vi "Segmentation.vi"(9 "sample time":dbl=1000.0, 11 "relative time":dbl[](array[numeric])=[1.0, 4.0, 7.0, 12.0, 15.0, 20.0, 31.0, 48.0, 59.0, 67.0, 96.0, 105.0, 121.0, 143.0, 144.0, 159.0, 171.0, 179.0, 185.0, 246.0] format="%#_10g") -> (1 "Segmentation":sgl[](array[numeric]), 2 "mean":dbl format="%0.2f", 3 "tau":dbl[](array[numeric]) format="%#_10g")   [LabVIEW 2015]
uses:
  <vilib>/Analysis/baseanly.llb/Mean (DBL).vi
  <vilib>/Analysis/NI_AALBase.lvlib
panel:
  out "Size in":i32
  out "index":sgl format="%#_10g"
  out "size segmentation":i32
  out "size tau":i32
  out "vector size":i32
  out "LsupLazo":sgl format="%#_10g"
  out "Datolazo":dbl format="%#_10g"
  out "Lsup":dbl format="%#_10g"
  out "dato":dbl format="%#_10g"
  out "Linf":dbl format="%#_10g"
  out "i vector":i32
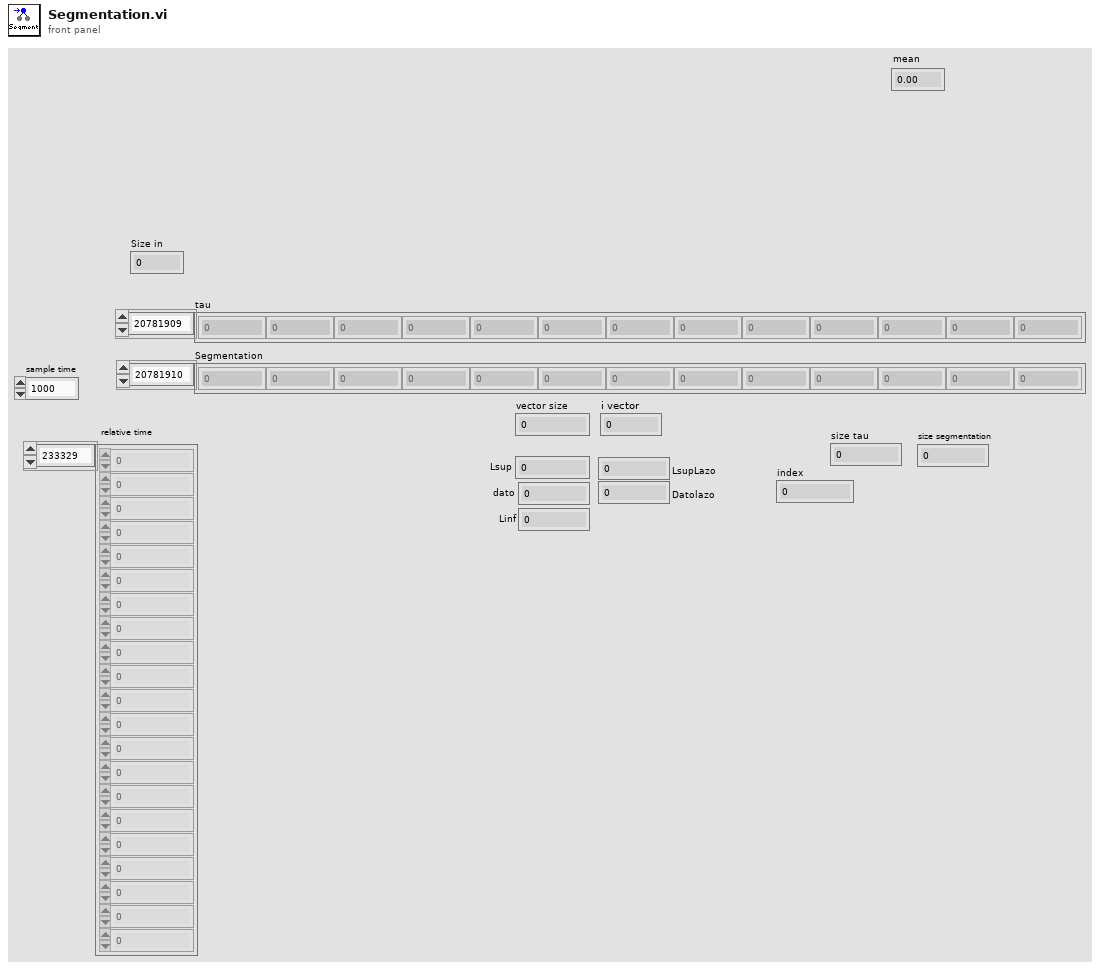
[diagram p1: front panel]
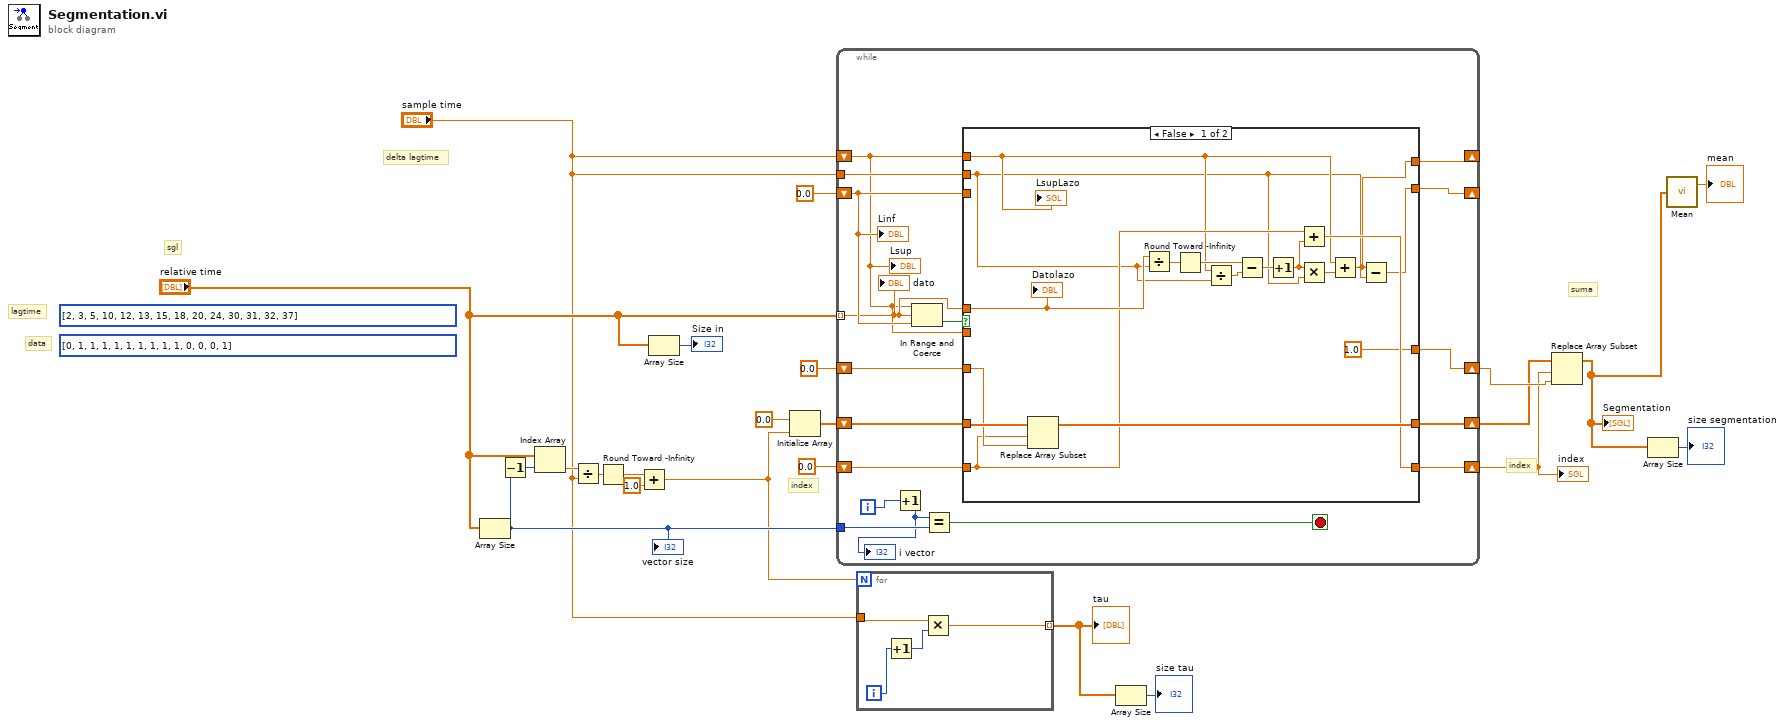
[diagram p0: block diagram]
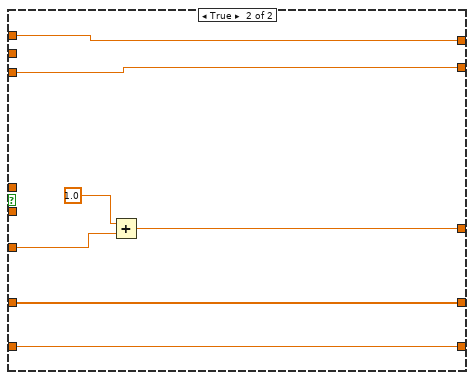
[diagram p2: hidden frame]
diagram:
  (unwired) i32[] [0, 1, 1, 1, 1, 1, 1, 1, 1, 1, 0, 0, 0, 1]
  (unwired) i32[] [2, 3, 5, 10, 12, 13, 15, 18, 20, 24, 30, 31, 32, 37]
  # "sgl"
  # "suma"
  # "index"
  # "index"
  # "delta lagtime"
  # "data"
  # "lagtime"
  n1 = Array Size(array="relative time") -> (size(s)=w18:i32)
  "vector size" <- w18
  n2 = Decrement(x=w18) -> (x-1=w16:i32)
  n3 = Index Array(array="relative time", index=w16) -> (element=w15:dbl)
  n4 = Divide(x=w15, y="sample time") -> (x/y=w19:dbl)
  n5 = Round Toward -Infinity(1:w19) -> (0:w14:dbl)
  n6 = Add(x=w14, y=sgl 1.0) -> (x+y=w12:dbl)
  n7 = Array Size(array="relative time") -> (size(s)=→"Size in":i32)
  n8 = Initialize Array(sgl 0.0 ("lower limit"), w12) -> (w21:sgl[])
  n9 = while {
    tunnel: "relative time" -> [w31] mode=indexing
    shift-right: [w26] -> w8
    shift-left: sgl 0.0 ("lower limit") -> [w39]
    shift-right: [w30] -> _
    shift-left: "sample time" -> [w28]
    tunnel: "sample time" -> [w29]
    shift-right: [w37] -> _
    shift-left: sgl 0.0 ("lower limit") -> [w38]
    tunnel: w18 -> [w36]
    shift-right: [w32] -> w6
    shift-left: w21 -> [w35]
    shift-right: [w33] -> w7
    shift-left: sgl 0.0 ("lower limit") -> [w34]
    i -> [w25]
    stop <- w27 stop-if-true
    n10 = Increment(x=w25) -> (x+1=w24:i32)
    "i vector" <- w24
    n11 = In Range and Coerce(upper limit=w28, x=w31, lower limit=w38) -> (In Range?=w40:bool)  [unwired: 1 out]
    n12 = Equal?(x=w24, y=w36) -> (x = y?=w27:bool)
    n13 = case shown="False" w40 {
      tunnel: [sgl 1.0 ("lower limit") w60] -> w26
      tunnel: w39 -> [w56 w64]
      tunnel: w28 -> [w46 w63]
      tunnel: [w44 w63] -> w30
      tunnel: w29 -> [w43 _]
      tunnel: w38 -> [_ w62]
      tunnel: [w42 w62] -> w37
      tunnel: w35 -> [w57 w59]
      tunnel: [w55 w59] -> w32
      tunnel: w34 -> [w49 w61]
      tunnel: [w48 w61] -> w33
      tunnel: w31 -> [w54 _]
      tunnel: w28 -> [_ _]
      frame False {
        n14 = Replace Array Subset(array=w57, new element=w56, index=w49) -> (w55:sgl[])
        n15 = Divide(x=w54, y=w43) -> (x/y=w53:dbl)
        n16 = Round Toward -Infinity(1:w53) -> (0:w52:dbl)
        n17 = Divide(x=w46, y=w43) -> (x/y=w51:dbl)
        n18 = Subtract(x=w52, y=w51) -> (x-y=w50:dbl)
        n19 = Increment(x=w50) -> (x+1=w47:dbl)
        n20 = Add(x=w49, y=w47) -> (x+y=w48:dbl)
        n21 = Multiply(x=w47, y=w43) -> (x*y=w45:dbl)
        n22 = Add(x=w46, y=w45) -> (x+y=w44:dbl)
        n23 = Subtract(x=w44, y=w43) -> (x-y=w42:dbl)
        "LsupLazo" <- w46
        "Datolazo" <- w54
      }
      frame True {
        n24 = Add(x=sgl 1.0 ("lower limit"), y=w64) -> (x+y=w60:sgl)
      }
    }
    "Lsup" <- w28
    "dato" <- w31
    "Linf" <- w38
  }
  "index" <- w7
  n25 = for {
    N: w12 -> [_]
    tunnel: "sample time" -> [w68]
    tunnel: [w65] -> w11 mode=indexing
    i -> [w66]
    n26 = Increment(x=w66) -> (x+1=w67:i32)
    n27 = Multiply(x=w68, y=w67) -> (x*y=w65:dbl)
  }
  "tau" <- w11
  n28 = Array Size(array=w11) -> (size(s)=→"size tau":i32)
  n29 = Replace Array Subset(array=w6, new element=w8, index=w7) -> (w3:sgl[])
  "Segmentation" <- w3
  n30 = Array Size(array=w3) -> (size(s)=→"size segmentation":i32)
  n31 = call-poly <vilib>:"Mean.vi"("X"=w3) -> ("mean"=→"mean":dbl)  [unwired: 1 out]
